vi "LoadTimingSettings.vi"(2 "error in (no error)":errorcluster, 3 "Time Card/Channels":i32[](array[numeric]), 4 "Tree DVR In":refnum<data-value>) -> (0 "error out":errorcluster, 1 "Timing Card Settings":T1[][](array[typedef]) {"FrontPanelTime" format="%.3p"; "Pulse width (s)" format="%.3p"; "Delay (s)" format="%.3p"})   [LabVIEW 2014]
uses:
  <vilib>/MDSplus/Classes/Tree_Class/Tree.lvclass
  Controls/TimingChannelSettings.ctl
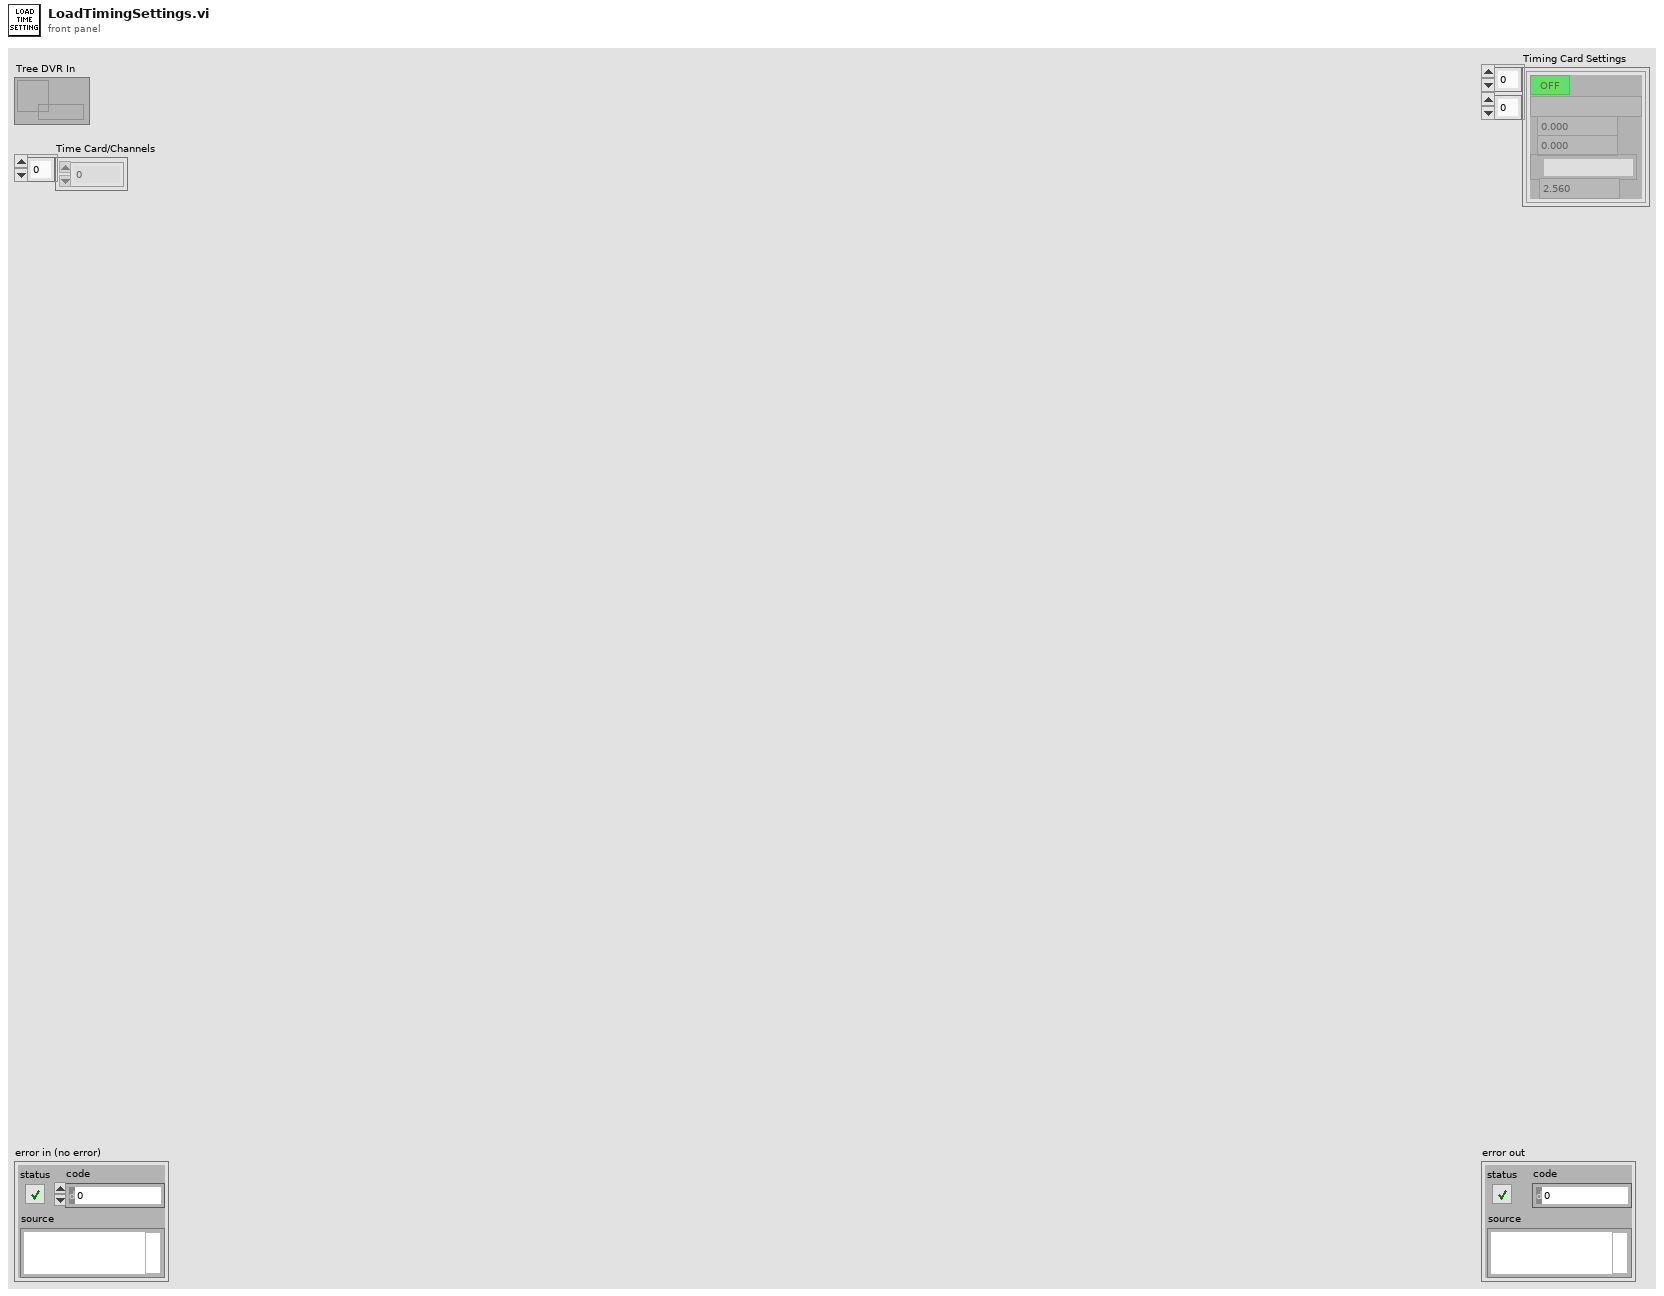
[diagram p1: front panel]
types:
  T1 = typedef "TimingChannelSettings.ctl" = cluster{"Delay (s)":dbl, "Pulse width (s)":dbl, "Active":bool, "Channel Name":string, "counter":tag, "FrontPanelTime":dbl}
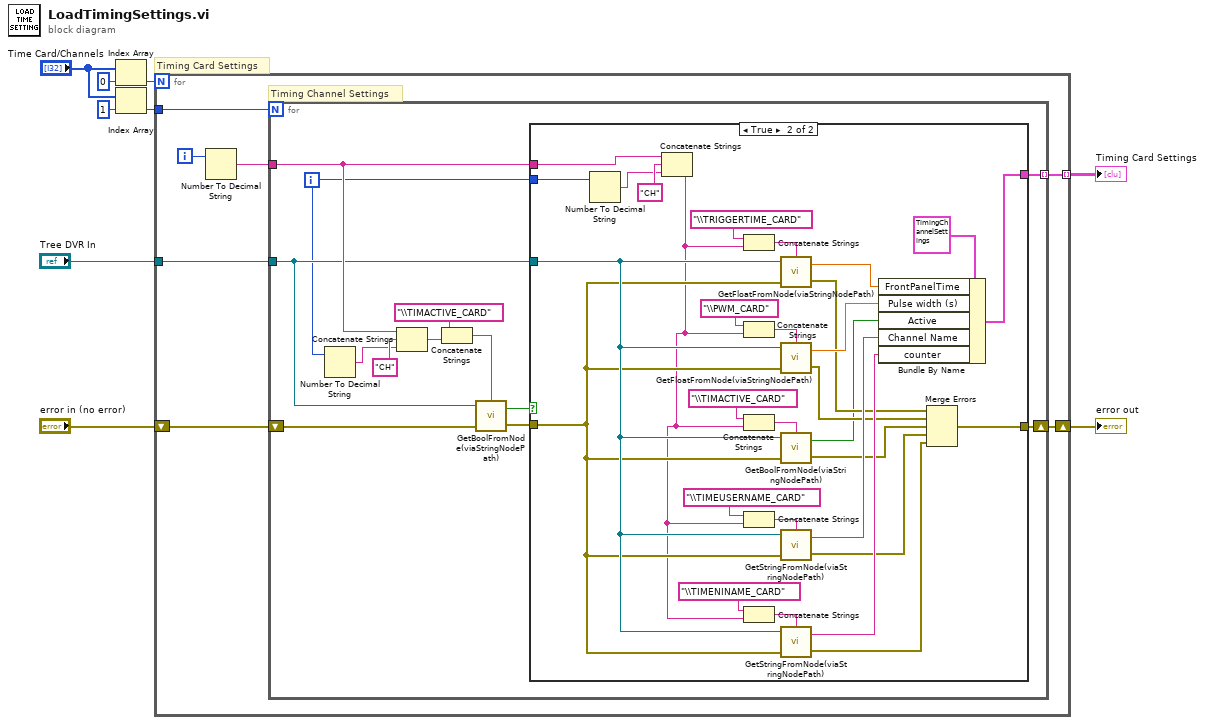
[diagram p0: block diagram]
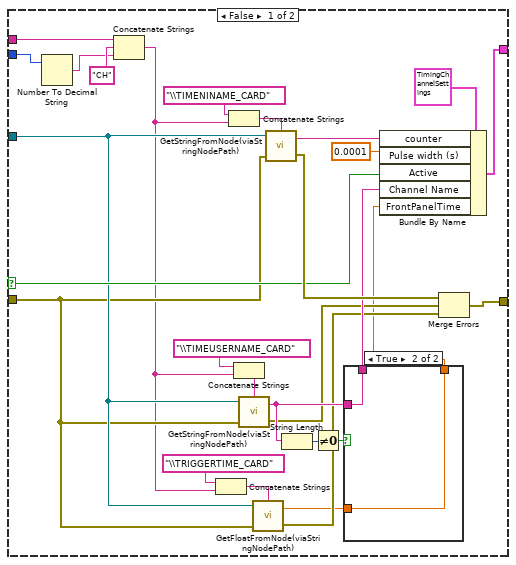
[diagram p2: hidden frame]
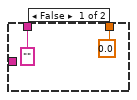
[diagram p3: hidden frame]
diagram:
  # "Timing Card Settings"
  n1 = Index Array(array="Time Card/Channels", index=0) -> (element=w6:i32)
  n2 = Index Array(array="Time Card/Channels", index=1) -> (element=w9:i32)
  n3 = for {
    N: w6 -> [_]
    tunnel: "Tree DVR In" -> [w16]
    tunnel: [w13] -> w1 mode=indexing
    shift-right: [w12] -> w2
    shift-left: "error in (no error)" -> [w11]
    tunnel: w9 -> [w10]
    i -> [w15]
    # "Timing Channel Settings"
    n4 = Number To Decimal String(number=w15) -> (decimal integer string=w14:string)  [unwired: 1 in]
    n5 = for {
      N: w10 -> [_]
      tunnel: w16 -> [w19]
      tunnel: w14 -> [w24]
      tunnel: [w29] -> w13 mode=indexing
      shift-right: [w28] -> w12
      shift-left: w11 -> [w21]
      i -> [w17]
      n6 = Number To Decimal String(number=w17) -> (decimal integer string=w26:string)  [unwired: 1 in]
      n7 = Concatenate Strings(w24, "CH" ("string"), w26) -> (w22:string)
      n8 = Concatenate Strings("\\TIMACTIVE_CARD" ("string"), w22) -> (w25:string)
      n9 = call "GetBoolFromNode(viaStringNodePath).vi"("Path"=w25, "error in"=w21, "Tree DVR in"=w19) -> ("error out"=w20:errorcluster, "Bool Out"=w18:bool)  [unwired: 1 in]
      n10 = case shown="True" w18 {
        selector: w18 -> [w44 _]
        tunnel: w19 -> [w36 w87]
        tunnel: w17 -> [w49 w86]
        tunnel: [w56 w71] -> w29
        tunnel: [w46 w70] -> w28
        tunnel: w20 -> [w35 w69]
        tunnel: w24 -> [w50 w65]
        frame False {
          n11 = Number To Decimal String(number=w49) -> (decimal integer string=w52:string)  [unwired: 1 in]
          n12 = Concatenate Strings(w50, "CH" ("string"), w52) -> (w30:string)
          n13 = Concatenate Strings("\\TRIGGERTIME_CARD" ("string"), w30) -> (w38:string)
          n14 = Concatenate Strings("\\TIMENINAME_CARD" ("string"), w30) -> (w54:string)
          n15 = Concatenate Strings("\\TIMEUSERNAME_CARD" ("string"), w30) -> (w47:string)
          n16 = call "GetStringFromNode(viaStringNodePath).vi"("Path"=w47, "error in"=w35, "Tree DVR in"=w36) -> ("error out"=w39:errorcluster, "String out"=w41:string)  [unwired: 1 in]
          n17 = call "GetFloatFromNode(viaStringNodePath).vi"("Path"=w38, "error in"=w35, "Tree DVR in"=w36) -> ("error out"=w34:errorcluster, "Float64"=w33:dbl)  [unwired: 1 in]
          n18 = call "GetStringFromNode(viaStringNodePath).vi"("Path"=w54, "error in"=w35, "Tree DVR in"=w36) -> ("error out"=w45:errorcluster, "String out"=w32:string)  [unwired: 1 in]
          n19 = String Length(string=w41) -> (length=w43:i32)
          n20 = Not Equal To 0?(x=w43) -> (x != 0?=w42:bool)
          n21 = case shown="True" w42 {
            tunnel: ["" w61] -> w40
            tunnel: w41 -> [_ w61]
            tunnel: w33 -> [_ w60]
            tunnel: [0.0 ("Float64") w60] -> w31
            frame False {
            }
            frame True {
            }
          }
          n22 = Bundle By Name(cluster=T1 {"Delay (s)"=0.0, "Pulse width (s)"=0.009999999776482582, "Active"=TRUE, "Channel Name"="Fiber 8", "counter"="PXI1Slot8/ctr7", "FrontPanelTime"=0.0} ("Counters"), "counter"=w32, "Pulse width (s)"=0.0001, "Active"=w44, "Channel Name"=w40, "FrontPanelTime"=w31) -> (w56:T1)
          n23 = Merge Errors(w45, w39, w34) -> (w46:errorcluster)
        }
        frame True {
          n24 = Number To Decimal String(number=w86) -> (decimal integer string=w66:string)  [unwired: 1 in]
          n25 = Concatenate Strings(w65, "CH" ("string"), w66) -> (w64:string)
          n26 = Concatenate Strings("\\TRIGGERTIME_CARD" ("string"), w64) -> (w85:string)
          n27 = Concatenate Strings("\\PWM_CARD" ("string"), w64) -> (w83:string)
          n28 = Concatenate Strings("\\TIMACTIVE_CARD" ("string"), w64) -> (w77:string)
          n29 = Concatenate Strings("\\TIMEUSERNAME_CARD" ("string"), w64) -> (w78:string)
          n30 = Concatenate Strings("\\TIMENINAME_CARD" ("string"), w64) -> (w79:string)
          n31 = call "GetFloatFromNode(viaStringNodePath).vi"("Path"=w85, "error in"=w69, "Tree DVR in"=w87) -> ("error out"=w76:errorcluster, "Float64"=w88:dbl)  [unwired: 1 in]
          n32 = call "GetFloatFromNode(viaStringNodePath).vi"("Path"=w83, "error in"=w69, "Tree DVR in"=w87) -> ("error out"=w75:errorcluster, "Float64"=w89:dbl)  [unwired: 1 in]
          n33 = call "GetBoolFromNode(viaStringNodePath).vi"("Path"=w77, "error in"=w69, "Tree DVR in"=w87) -> ("error out"=w74:errorcluster, "Bool Out"=w68:bool)  [unwired: 1 in]
          n34 = call "GetStringFromNode(viaStringNodePath).vi"("Path"=w78, "error in"=w69, "Tree DVR in"=w87) -> ("error out"=w73:errorcluster, "String out"=w90:string)  [unwired: 1 in]
          n35 = call "GetStringFromNode(viaStringNodePath).vi"("Path"=w79, "error in"=w69, "Tree DVR in"=w87) -> ("error out"=w72:errorcluster, "String out"=w91:string)  [unwired: 1 in]
          n36 = Bundle By Name(cluster=T1 {"Delay (s)"=0.0, "Pulse width (s)"=0.009999999776482582, "Active"=TRUE, "Channel Name"="Fiber 8", "counter"="PXI1Slot8/ctr7", "FrontPanelTime"=0.0} ("Counters"), "FrontPanelTime"=w88, "Pulse width (s)"=w89, "Active"=w68, "Channel Name"=w90, "counter"=w91) -> (w71:T1)
          n37 = Merge Errors(w76, w75, w74, w73, w72) -> (w70:errorcluster)
        }
      }
    }
  }
  "error out" <- w2
  "Timing Card Settings" <- w1
